vi "Load port config.vi"(8 "error in (no error)":errorcluster) -> (0 "error out":errorcluster, 3 "Comm ports out":T1={"Piezo driver"="COM2", "Cam Session"="", "Arduino"="COM2"})   [LabVIEW 2020]
uses:
  <vilib>/Utility/config.llb/NI_LVConfig.lvlib
  <vilib>/Utility/config.llb/Read Key (String).vi
  <vilib>/userDefined/High Color/IMAQdx.ctl
  Controls/Communication ports ---typedef.ctl
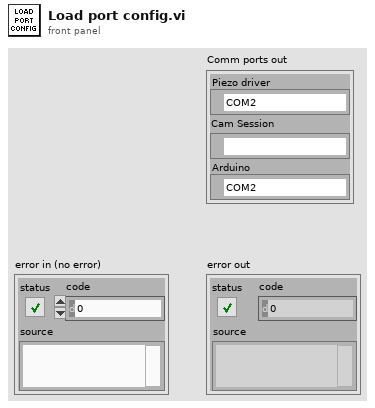
[diagram p1: front panel]
types:
  T1 = typedef "Communication ports ---typedef.ctl" = cluster{"Piezo driver":refnum<visa-resource-name>, "Cam Session":T2, "Arduino":refnum<visa-resource-name>}
  T2 = typedef "IMAQdx.ctl" = refnum<k21>
  T3 = typedef "NI_LVConfig.lvlib/Config Data RefNum.ctl" = refnum<k1>
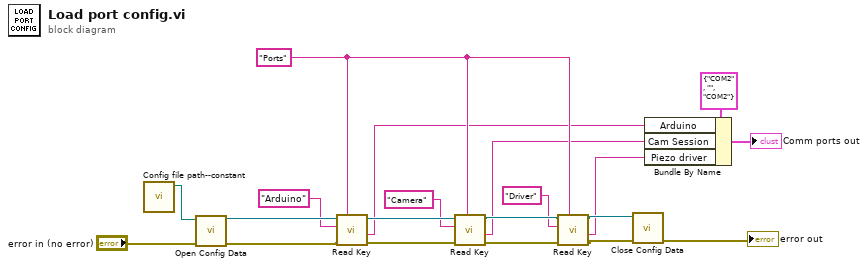
[diagram p0: block diagram]
diagram:
  w11 = "Ports" ("section")
  n1 = call "Config file path--constant.vi"() -> ("appended path"=w20:path)  [unwired: 11 in]
  n2 = call <vilib>:"Open Config Data.vi"("error in (no error)"="error in (no error)", "configuration file path"=w20) -> ("error out"=w17:errorcluster, "refnum"=w16:T3)  [unwired: 7 in, 1 out]
  n3 = call-poly <vilib>:"Read Key.vi"("section"=w11, "error in (no error)"=w17, "key"="Arduino", "refnum"=w16) -> ("error out"=w13:errorcluster, "value"=w3:string, "refnum out"=w14:T3)  [unwired: 4 in, 1 out]
  n4 = call-poly <vilib>:"Read Key.vi"("section"=w11, "error in (no error)"=w13, "key"="Camera", "refnum"=w14) -> ("error out"=w10:errorcluster, "value"=w2:string, "refnum out"=w8:T3)  [unwired: 4 in, 1 out]
  n5 = call-poly <vilib>:"Read Key.vi"("section"=w11, "error in (no error)"=w10, "key"="Driver", "refnum"=w8) -> ("error out"=w9:errorcluster, "value"=w1:string, "refnum out"=w7:T3)  [unwired: 4 in, 1 out]
  n6 = call <vilib>:"Close Config Data.vi"("error in (no error)"=w9, "refnum"=w7) -> ("error out"=→"error out":errorcluster)  [unwired: 8 in, 1 out]
  n7 = Bundle By Name(cluster=T1 {"Piezo driver"="COM2", "Cam Session"="", "Arduino"="COM2"} ("Comm ports out"), "Arduino"=w3, "Cam Session"=w2, "Piezo driver"=w1) -> (→"Comm ports out":T1)
